vi "Read Data.vi"(8 "Error In":errorcluster, 11 "VISA IN":refnum<visa-resource-name>) -> (0 "Error Out":errorcluster, 1 "Output 2":string, 2 "Capacitance(pF)":string, 3 "VISA Out":refnum<visa-resource-name>, 4 "CAP (pF)":dbl)   [LabVIEW 2017]
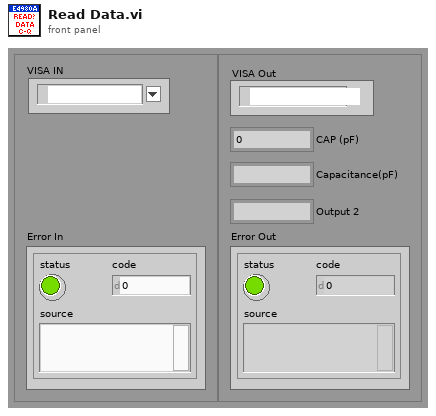
[diagram p1: front panel]
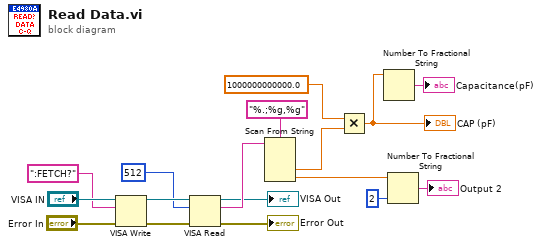
[diagram p0: block diagram]
diagram:
  n1 = VISA Write(VISA resource name="VISA IN", write buffer=":FETCH?", error in (no error)="Error In") -> (VISA resource name out=w14:refnum<visa-resource-name>, error out=w13:errorcluster)  [unwired: 1 out]
  n2 = VISA Read(VISA resource name=w14, byte count=u32 512, error in (no error)=w13) -> (VISA resource name out=→"VISA Out":refnum<visa-resource-name>, read buffer=w11:string, error out=→"Error Out":errorcluster)  [unwired: 1 out]
  n3 = Scan From String(format string="%.;%g,%g", input string=w11) -> (output 1=w7:dbl, output 2=w3:dbl)  [unwired: 4 in, 3 out]
  n4 = Multiply(x=1000000000000.0, y=w7) -> (x*y=w5:dbl)
  "CAP (pF)" <- w5
  n5 = Number To Fractional String(number=w5) -> (F-format string=→"Capacitance(pF)":string)  [unwired: 3 in]
  n6 = Number To Fractional String(number=w3, precision (6)=i16 2) -> (F-format string=→"Output 2":string)  [unwired: 2 in]
